vi "PUMP CONTROL.vi"() -> ()   [LabVIEW 2012]
uses:
  <vilib>/Instr/_visa.llb/VISA Configure Serial Port (Instr).vi
panel:
  out "return count":u32
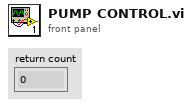
[diagram p1: front panel]
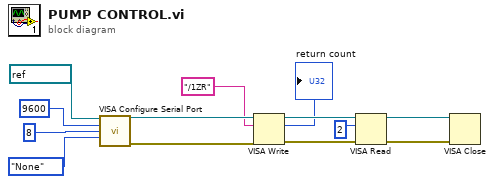
[diagram p0: block diagram]
diagram:
  n1 = call-poly "VISA Configure Serial Port"("VISA resource name"=refnum<visa-resource-name> "COM4", "baud rate (9600)"=u32 9600, "data bits (8)"=u16 8, "parity (0:none)"=enum16{"None", "Odd", "Even", "Mark", "Space"}."None") -> ("VISA resource name out"=w9:refnum<visa-resource-name>, "error out"=w7:errorcluster)  [unwired: 10 in]
  n2 = VISA Write(VISA resource name=w9, write buffer="/1ZR", error in (no error)=w7) -> (VISA resource name out=w6:refnum<visa-resource-name>, return count=→"return count":u32, error out=w5:errorcluster)
  n3 = VISA Read(VISA resource name=w6, byte count=u32 2, error in (no error)=w5) -> (VISA resource name out=w4:refnum<visa-resource-name>, error out=w3:errorcluster)  [unwired: 2 out]
  n4 = VISA Close(VISA resource name=w4, error in (no error)=w3) -> ()  [unwired: 1 out]
